vi "AutoWait.vi"(8 "error in (no error)":errorcluster, 11 "TimeOut (s)":dbl) -> (0 "error out":errorcluster)   [LabVIEW 2020]
doc: "Wrapper class for auto do nothing and wait\nInput:\n -- error in -- Cluster \n -- time out -- Double -- how long to wait B4 quitting\nOutput:\n -- error out -- Cluster"
uses:
  <vilib>/Utility/semaphor.llb/Obtain Semaphore Reference.vi
  <vilib>/Rock Robotics/WPI/ThirdParty/JAS_Junk/TrajLib/Timer_Reset.vi
  <vilib>/Rock Robotics/WPI/ThirdParty/JAS_Junk/TrajLib/Trajectory_Library.lvlib
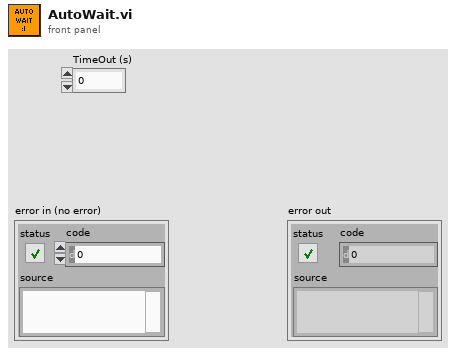
[diagram p1: front panel]
types:
  T1 = typedef "Trajectory_Library.lvlib/TIMER.ctl" = cluster{"StartTime":dbl, "Accumulated TIme":dbl, "Running":bool, "semaphore":T2}
  T2 = typedef "Semaphore RefNum" = refnum<k1>
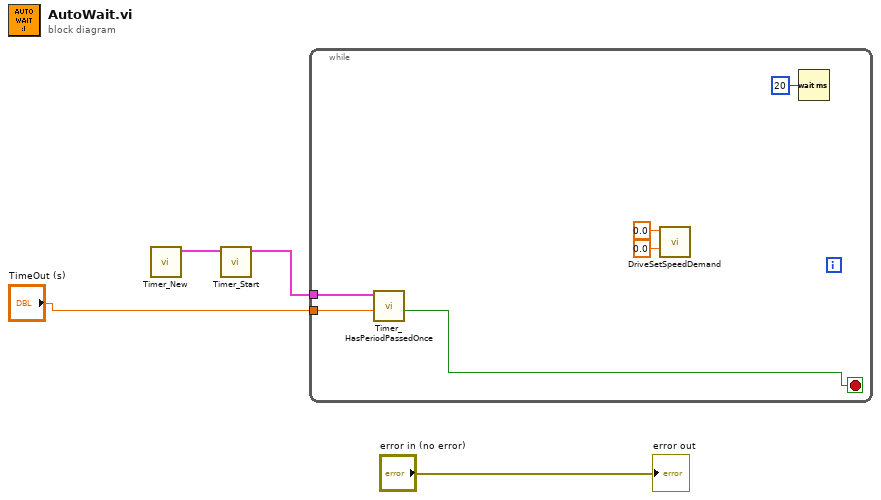
[diagram p0: block diagram]
diagram:
  n1 = call <vilib>:"Timer_New.vi"() -> ("TIMER"=w3:T1)  [unwired: 11 in]
  n2 = call <vilib>:"Timer_Start.vi"("in Timer"=w3) -> ("out Timer"=w2:T1)  [unwired: 10 in]
  n3 = while {
    tunnel: w2 -> [w10]
    tunnel: "TimeOut (s)" -> [w9]
    stop <- w5 stop-if-true
    n4 = call <vilib>:"Timer_HasPeriodPassedOnce.vi"("Period"=w9, "in Timer"=w10) -> ("Expired"=w5:bool)  [unwired: 7 in, 2 out]
    n5 = call "DriveSetSpeedDemand.vi"("RSpeedDemand (ft/s)"=0.0, "LSpeedDemand (ft/s)"=0.0) -> ()  [unwired: 10 in]
    n6 = Wait (ms)(milliseconds to wait=u32 20) -> ()  [unwired: 1 out]
  }
  "error out" <- "error in (no error)"
